vi "resolveEmbeddedTypes.vi"(1 "Message Definition":string) -> (0 "Md5 Text":string)   [LabVIEW 2010]
panel:
  # "Any primitive types are kept the same\nNon primitive type fields are replaced with\nthe md5 hash of their message"
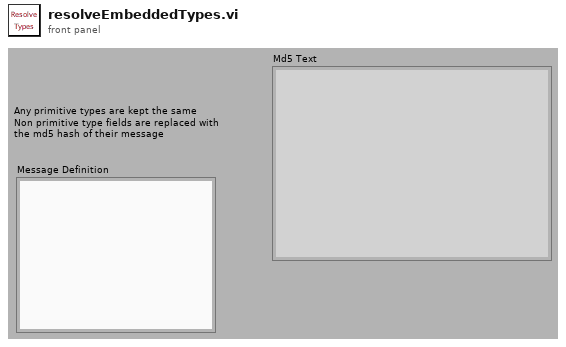
[diagram p1: front panel]
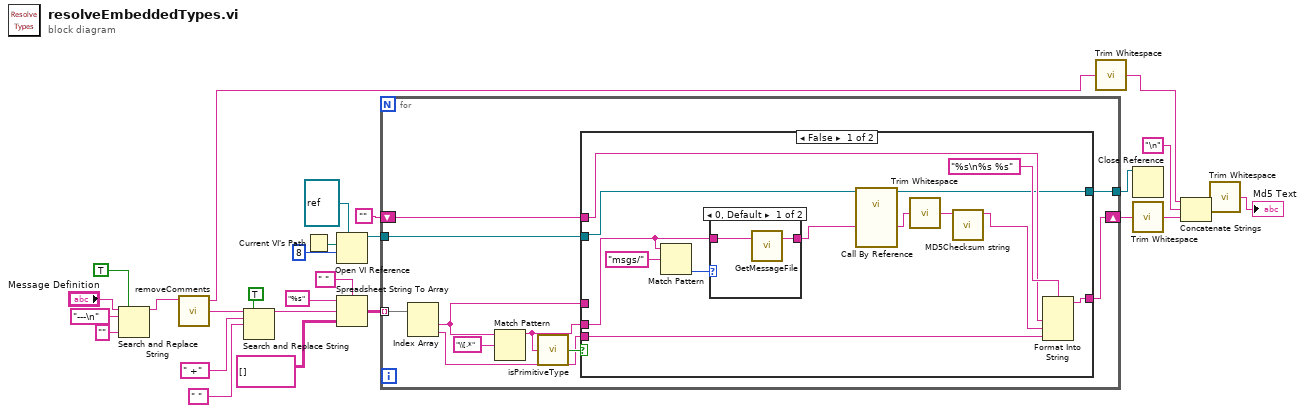
[diagram p0: block diagram]
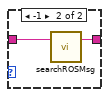
[diagram p2: hidden frame]
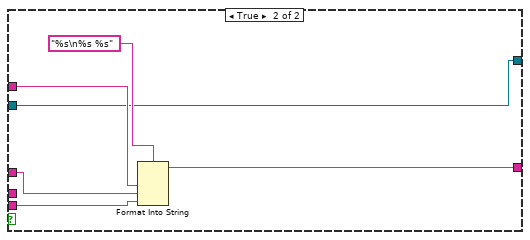
[diagram p3: hidden frame]
diagram:
  n1 = Search and Replace String(replace all?=TRUE ("replace all? (F)"), input string="Message Definition", search string="---\n", replace string="" ("replace string (\"\")")) -> (result string=w8:string)  [unwired: 4 in, 3 out]
  n2 = call "removeComments.vi"("String"=w8) -> ("Body"=w12:string, "Constants"=w4:string)  [unwired: 3 in, 1 out]
  n3 = Search and Replace String(replace all?=TRUE ("replace all? (F)"), input string=w12, search string=" +", replace string=" " ("search string")) -> (result string=w20:string)  [unwired: 4 in, 3 out]
  n4 = Current VI's Path() -> (path=w13:path)
  n5 = Open VI Reference(type specifier VI Refnum (for type only)=refnum<vi> refnum, vi path=w13, options=8) -> (vi reference=w15:refnum<vi>)  [unwired: 3 in, 1 out]
  n6 = Spreadsheet String To Array(delimiter (Tab)=" " ("regular expression"), format string="%s", spreadsheet string=w20, array type (2D Dbl)=string[][] []) -> (array=w21:string[][])
  n7 = for {
    tunnel: w21 -> [w37] mode=indexing
    shift-right: [w33] -> w18
    shift-left: "" -> [w35]
    tunnel: w15 -> [w31]
    tunnel: [w30] -> w14
    n8 = Index Array(array=w37) -> (element #1=w28:string, element #2=w34:string)  [unwired: 2 in]
    n9 = Match Pattern(string=w28, regular expression="\\[.*") -> (before substring=w29:string)  [unwired: 1 in, 3 out]
    n10 = call "isPrimitiveType.vi"("field type"=w29) -> ("Boolean"=w36:bool)
    n11 = case shown="False" w36 {
      tunnel: w35 -> [w46 w59]
      tunnel: w29 -> [w48 _]
      tunnel: w34 -> [w44 w58]
      tunnel: [w45 w57] -> w33
      tunnel: w31 -> [w43 w56]
      tunnel: [w42 w56] -> w30
      tunnel: w28 -> [_ w55]
      frame False {
        n12 = Match Pattern(string=w48, regular expression="msgs/") -> (offset past match=w49:i32)  [unwired: 1 in, 3 out]
        n13 = case shown="0, Default" w49 {
          tunnel: w48 -> [w52 w54]
          tunnel: [w51 w53] -> w41
          frame 0, Default {
            n14 = call "GetMessageFile.vi"("type"=w52) -> ("File"=w51:string)  [unwired: 1 in, 1 out]
          }
          frame -1 {
            n15 = call "searchROSMsg.vi"("type"=w54) -> ("File"=w53:string)  [unwired: 1 in, 1 out]
          }
        }
        n16 = call-by-ref "?"(reference=w43, "Body"=w41) -> (reference out=w42:refnum<vi>, "String"=w40:string)  [unwired: 1 in, 1 out]
        n17 = call <vilib>:"Trim Whitespace.vi"("string"=w40) -> ("trimmed string"=w39:string)  [unwired: 1 in]
        n18 = call <vilib>:"MD5Checksum string.vi"("Message String"=w39) -> ("MD5 message-digest"=w38:string)  [unwired: 10 in]
        n19 = Format Into String(format string="%s\n%s %s", w46, w38, w44) -> (resulting string=w45:string)  [unwired: 2 in, 1 out]
      }
      frame True {
        n20 = Format Into String(format string="%s\n%s %s", w59, w55, w58) -> (resulting string=w57:string)  [unwired: 2 in, 1 out]
      }
    }
  }
  n21 = call <vilib>:"Trim Whitespace.vi"("string"=w4) -> ("trimmed string"=w3:string)  [unwired: 1 in]
  n22 = Close Reference(reference=w14) -> ()  [unwired: 1 in, 1 out]
  n23 = call <vilib>:"Trim Whitespace.vi"("string"=w18) -> ("trimmed string"=w11:string)  [unwired: 1 in]
  n24 = Concatenate Strings(w3, "\n" ("string"), w11) -> (w2:string)
  n25 = call <vilib>:"Trim Whitespace.vi"("string"=w2) -> ("trimmed string"=→"Md5 Text":string)  [unwired: 1 in]
